vi "toXml.vi"(8 "error in (no error)":errorcluster, 11 "RampEvent in":refnum<class "RampEvent.lvclass">) -> (0 "error out":errorcluster, 2 "scriptEventXML":refnum<class "xmlNode.lvclass">, 3 "RampEvent out":refnum<class "RampEvent.lvclass">)   [LabVIEW 2009, in "Tools.lvlib" / "Scripting.lvlib" / "RampEvent.lvclass"]
uses:
  RampEvent.lvclass
  xmlNode/xmlNode.lvclass
  DatabaseHelpers/Database Objects/Channel/Channel.lvclass
  ScriptEvent.lvclass
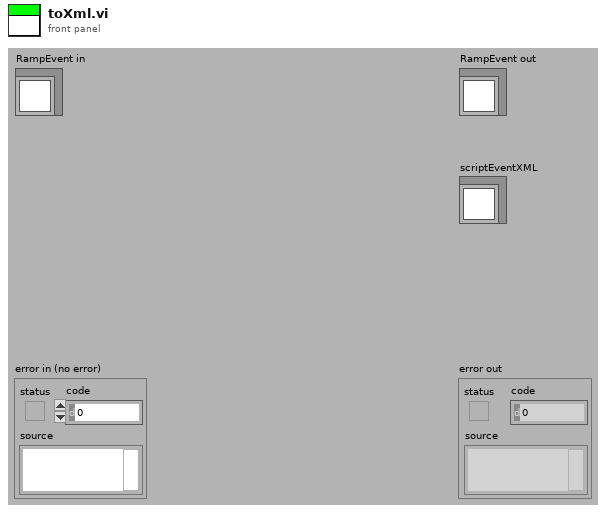
[diagram p1: front panel]
types:
  T1 = cluster{"attributeName":string, "channel_name":string}
  T2 = cluster{"attributeName":string, "channel_name":string}[]
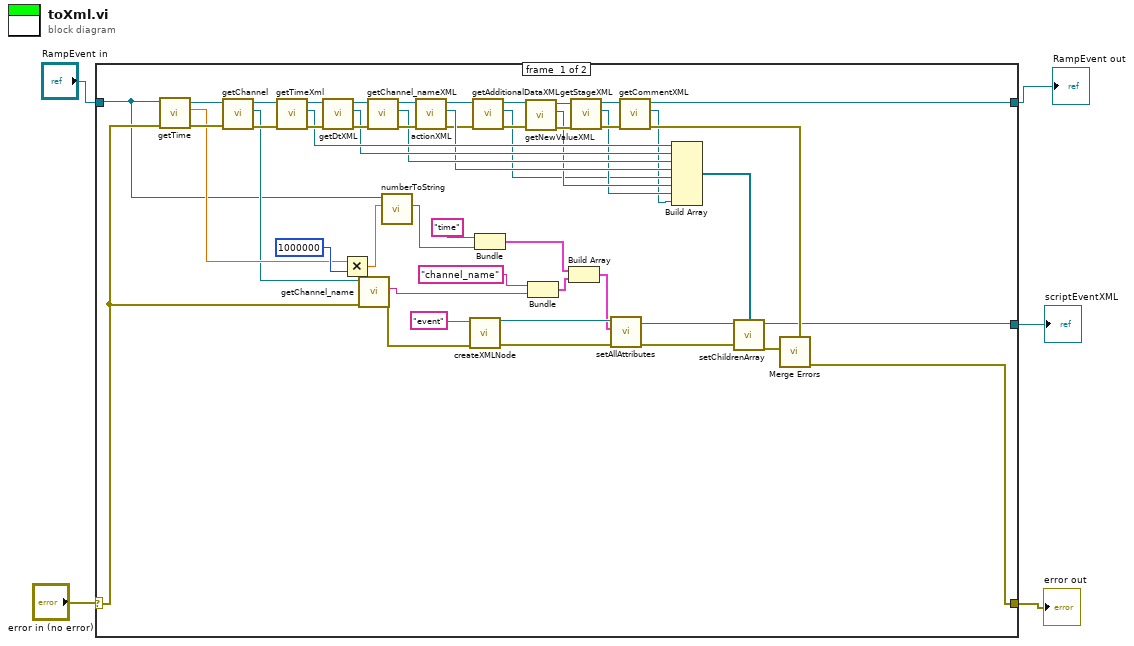
[diagram p0: block diagram]
diagram:
  n1 = case shown="No Error" "error in (no error)" {
    selector: "error in (no error)" -> [w16 w58]
    tunnel: "RampEvent in" -> [w8 w57]
    tunnel: [w24 w57] -> w3
    tunnel: [w15 w58] -> w2
    tunnel: [w23 _] -> w1
    frame #0 {
      n2 = call "getTime.vi"("error in (no error)"=w16, "ScriptEvent.lvclass in"=w8) -> ("error out"=w21:errorcluster, "time"=w18:dbl, "ScriptEvent.lvclass out"=w19:refnum<class "RampEvent.lvclass">)  [unwired: 7 in]
      n3 = call-dynamic "getChannel.vi"("error in (no error)"=w21, "ScriptEvent.lvclass in"=w19) -> ("error out"=w22:errorcluster, "Channel.lvclass"=w17:refnum<class "Channel.lvclass">, "ScriptEvent.lvclass out"=w20:refnum<class "RampEvent.lvclass">)  [unwired: 7 in]
      n4 = call "getTimeXml.vi"("error in (no error)"=w22, "ScriptEvent in"=w20) -> ("error out"=w54:errorcluster, "timeXML"=w44:refnum<class "xmlNode.lvclass">, "ScriptEvent out"=w49:refnum<class "RampEvent.lvclass">)  [unwired: 7 in]
      n5 = call "getDtXML.vi"("error in (no error)"=w54, "ScriptEvent in"=w49) -> ("error out"=w53:errorcluster, "dtXML"=w43:refnum<class "xmlNode.lvclass">, "ScriptEvent out"=w48:refnum<class "RampEvent.lvclass">)  [unwired: 7 in]
      n6 = Multiply(x=w18, y=1000000) -> (x*y=w7:dbl)
      n7 = call "getChannel_name.vi"("error in (no error)"=w16, "Channel.lvclass in"=w17) -> ("error out"=w55:errorcluster, "channel_name"=w33:string)  [unwired: 7 in, 1 out]
      n8 = call "getChannel_nameXML.vi"("error in (no error)"=w53, "ScriptEvent in"=w48) -> ("error out"=w52:errorcluster, "channel_nameXML"=w42:refnum<class "xmlNode.lvclass">, "ScriptEvent out"=w47:refnum<class "RampEvent.lvclass">)  [unwired: 7 in]
      n9 = call "numberToString.vi"("Numeric"=w7, "ScriptEvent in"=w8) -> ("String"=w6:string)  [unwired: 7 in, 2 out]
      n10 = call "actionXML.vi"("error in (no error)"=w52, "ScriptEvent in"=w47) -> ("error out"=w12:errorcluster, "actionXml"=w41:refnum<class "xmlNode.lvclass">, "ScriptEvent out"=w14:refnum<class "RampEvent.lvclass">)  [unwired: 7 in]
      n11 = call "createXMLNode.vi"("error in (no error)"=w55, "name"="event") -> ("error out"=w28:errorcluster, "xmlNode out"=w32:refnum<class "xmlNode.lvclass">)  [unwired: 8 in]
      n12 = call-dynamic "getAdditionalDataXML.vi"("error in (no error)"=w12, "RampEvent in"=w14) -> ("error out"=w11:errorcluster, "additionalDataXML"=w10:refnum<class "xmlNode.lvclass">, "RampEvent out"=w13:refnum<class "RampEvent.lvclass">)  [unwired: 7 in]
      n13 = Bundle("attributeName"="time", "String"=w6) -> (w31:cluster{"attributeName":string, "String":string})  [unwired: 1 in]
      n14 = call-dynamic "getNewValueXML.vi"("error in (no error)"=w11, "RampEvent in"=w13) -> ("error out"=w51:errorcluster, "newValueXML"=w40:refnum<class "xmlNode.lvclass">, "RampEvent out"=w46:refnum<class "RampEvent.lvclass">)  [unwired: 7 in]
      n15 = Bundle("attributeName"="channel_name", "channel_name"=w33) -> (w30:T1)  [unwired: 1 in]
      n16 = Build Array(w31, w30) -> (w29:T2)
      n17 = call "getStageXML.vi"("error in (no error)"=w51, "ScriptEvent in"=w46) -> ("error out"=w50:errorcluster, "stageXML"=w39:refnum<class "xmlNode.lvclass">, "ScriptEvent out"=w45:refnum<class "RampEvent.lvclass">)  [unwired: 7 in]
      n18 = call-dynamic "setAllAttributes.vi"("error in (no error)"=w28, "attributes"=w29, "xmlNode in"=w32) -> ("error out"=w27:errorcluster, "xmlNode out"=w26:refnum<class "xmlNode.lvclass">)  [unwired: 7 in]
      n19 = call "getCommentXML.vi"("error in (no error)"=w50, "ScriptEvent in"=w45) -> ("error out"=w37:errorcluster, "commentXML"=w9:refnum<class "xmlNode.lvclass">, "ScriptEvent out"=w24:refnum<class "RampEvent.lvclass">)  [unwired: 7 in]
      n20 = Build Array(w44, w43, w42, w41, w10, w40, w39, w9) -> (w38:refnum<class "xmlNode.lvclass">[])
      n21 = call-dynamic "setChildrenArray.vi"("error in (no error)"=w27, "Children"=w38, "xmlNode.lvclass in"=w26) -> ("error out"=w36:errorcluster, "xmlNode.lvclass out"=w23:refnum<class "xmlNode.lvclass">)  [unwired: 7 in]
      n22 = call <vilib>:"Merge Errors.vi"("error in 2 (no error)"=w36, "error in 1 (no error)"=w37) -> ("error out"=w15:errorcluster)  [unwired: 5 in]
    }
    frame #1 {
    }
  }
  "error out" <- w2
  "RampEvent out" <- w3
  "scriptEventXML" <- w1
